vi "Session Write.vi"(8 "error in (no error)":errorcluster, 9 "Timeout":i32=5000, 10 "Message Packet In":T1, 11 "HSMS Class in":refnum<class "HSMS Class.lvclass">) -> (0 "error out":errorcluster, 2 "Message Packet Out":T1, 3 "HSMS Class out":refnum<class "HSMS Class.lvclass">)   [LabVIEW 2020, in "SECS Communication.lvlib" / "HSMS Class.lvclass"]
uses:
  HSMS Class.lvclass
  Message Packet.ctl
  HSMS Class.lvclass/HSMS Class.ctl
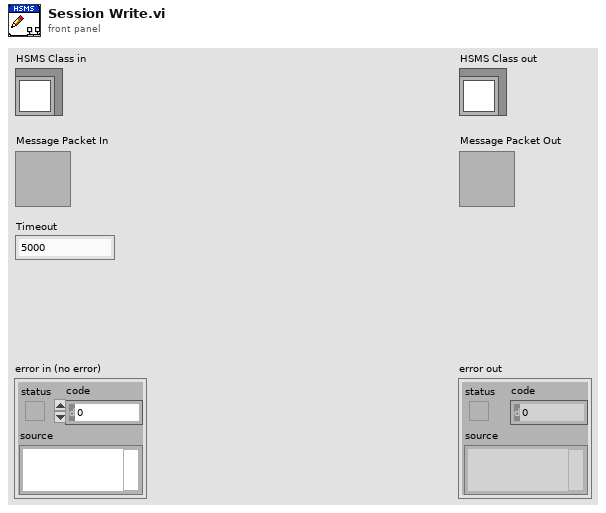
[diagram p1: front panel]
types:
  T1 = typedef "SECS Communication.lvlib/HSMS Class.lvclass/Message Packet.ctl" = cluster{"Message Header Cluster":T2, "Message Header":u8[], "Message Text":u8[]}
  T2 = typedef "SECS Communication.lvlib/HSMS Class.lvclass/Message Header.ctl" = cluster{"Byte 0-1(Session ID)":u16, "W-Bit":bool, "Byte 2":u8, "Byte 3":u8, "Byte 4(PType)":T3, "Byte 5(SType)":T4, "Byte 6-9(System Btyes)":u8[]}
  T3 = typedef "SECS Communication.lvlib/HSMS Class.lvclass/PType.ctl" = enum8{"SECS-II Encoding", "Reserved"}
  T4 = typedef "SECS Communication.lvlib/HSMS Class.lvclass/SType.ctl" = enum8{"Data Message", "Select.req", "Select.rsp", "Deselect.req", "Deselect.rsp", "Linktest.req", "Linktest.rsp", "Reject.req", "Separate.req"}
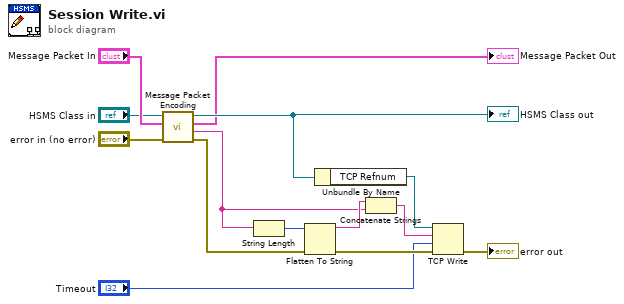
[diagram p0: block diagram]
diagram:
  n1 = call "Message Packet Encoding.vi"("error in (no error)"="error in (no error)", "Message Packet In"="Message Packet In", "HSMS Class in"="HSMS Class in") -> ("error out"=w7:errorcluster, "Data"=w4:string, "Message Packet Out"=→"Message Packet Out":T1, "HSMS Class out"=w2:refnum<class "HSMS Class.lvclass">)  [unwired: 5 in]
  "HSMS Class out" <- w2
  n2 = String Length(string=w4) -> (length=w14:i32)
  n3 = Flatten To String(anything=w14, error in (no error)=w7) -> (data string=w13:string, error out=w11:errorcluster)  [unwired: 3 out]
  n4 = Unbundle By Name(w2) -> ("TCP Refnum"=w9:refnum<k5>)
  n5 = Concatenate Strings(w13, w4) -> (w12:string)
  n6 = TCP Write(connection ID=w9, data in=w12, error in (no error)=w11, 9:"Timeout") -> (error out=→"error out":errorcluster)  [unwired: 2 out]
